vi "Destroy.vi"(0 "Suggestion IO in":refnum<class "Static Listbox IO.lvclass">, 11 "error in (no error)":errorcluster) -> (4 "Suggestion IO out":refnum<class "Static Listbox IO.lvclass">, 15 "error out":errorcluster)   [LabVIEW 2016, in "Static Listbox IO.lvclass"]
uses:
  Static Listbox IO.lvclass
  Static Listbox IO.lvclass/Static Listbox IO.ctl
  base/SuggestionIObase.lvclass
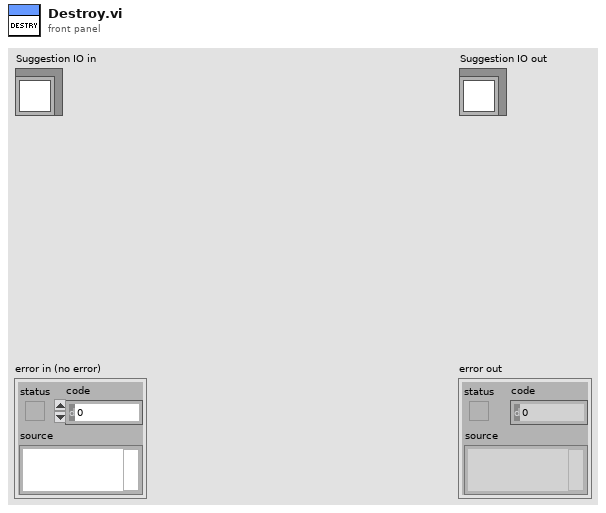
[diagram p1: front panel]
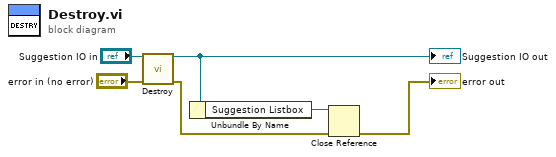
[diagram p0: block diagram]
diagram:
  n1 = call-parent "Destroy.vi"("Suggestion IO in"="Suggestion IO in", "error in (no error)"="error in (no error)") -> ("Suggestion IO out"=w4:refnum<class "Static Listbox IO.lvclass">, "error out"=w2:errorcluster)  [unwired: 12 in]
  "Suggestion IO out" <- w4
  n2 = Unbundle By Name(w4) -> ("Suggestion Listbox"=w3:refnum<vi>)
  n3 = Close Reference(reference=w3, error in (no error)=w2) -> (error out=→"error out":errorcluster)
